vi "add set lengtou2 position(SubVI).vi"(9 "字符串":string) -> (0 "布尔 3":bool, 2 "连接的字符串":string)   [LabVIEW 2019]
panel:
  in  "cancel":bool
  in  "ok":bool
  in  "Position":dbl=2.0 min=0.0 max=400.0
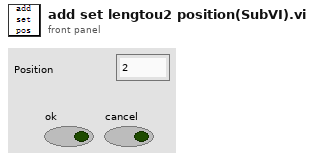
[diagram p1: front panel]
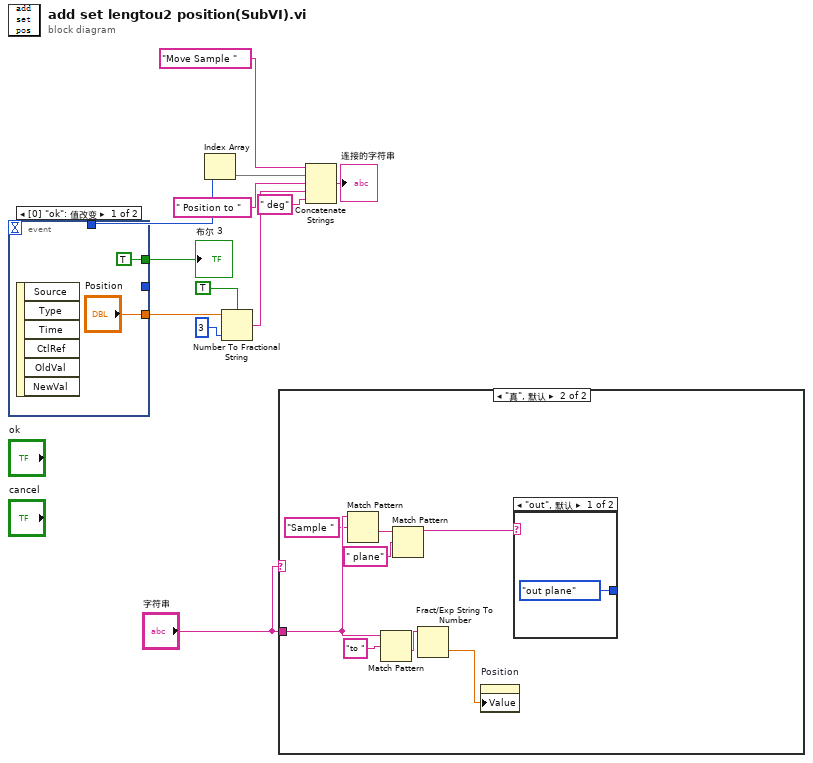
[diagram p0: block diagram]
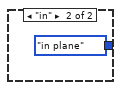
[diagram p3: hidden frame]
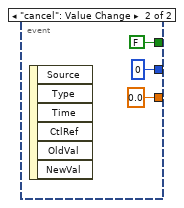
[diagram p4: hidden frame]
diagram:
  n1 = event shown="[0] \"ok\": 值改变" {
    selector: _ -> [_ _]
    dyn-events: _ -> [_ _]
    timeout: _ -> [_ _]
    tunnel: [_ 0 ("Rate输入")] -> _
    tunnel: ["Position" 0.0 ("Field")] -> w12
    tunnel: [TRUE FALSE] -> w13
    tunnel: [w14 _] -> w1
    event "ok": Value Change {
      n2 = event-data() -> ()  [unwired: 1 in, 6 out]
    }
    event "cancel": Value Change {
      n3 = event-data() -> ()  [unwired: 1 in, 6 out]
    }
  }
  "布尔 3" <- w13
  n4 = Index Array(index=w1) -> (array=w6:string[], element=w3)
  n5 = Number To Fractional String(use system decimal point (T)=TRUE ("使用系统小数点(T)"), number=w12, precision (6)=i16 3 ("精度(6)")) -> (F-format string=w10:string)  [unwired: 1 in]
  n6 = case shown="\"真\", 默认" "字符串" {
    tunnel: "字符串" -> [_ w26]
    frame "" {
    }
    frame "真", Default {
      n7 = Match Pattern(string=w26, regular expression="Sample " ("正则表达式")) -> (after substring=w23:string)  [unwired: 1 in, 3 out]
      n8 = Match Pattern(string=w26, regular expression="to " ("正则表达式")) -> (after substring=w28:string)  [unwired: 1 in, 3 out]
      n9 = Match Pattern(string=w23, regular expression=" plane" ("正则表达式")) -> (before substring=w22:string)  [unwired: 1 in, 3 out]
      n10 = Fract/Exp String To Number(string=w28) -> (number=w20:dbl)  [unwired: 3 in, 1 out]
      n11 = property on="Position" class="DigNum (严格)"("Value"=w20) -> ()  [unwired: 2 in, 2 out]
      n12 = case shown="\"out\", 默认" w22 {
        tunnel: [enum16{"in plane", "out plane"}."out plane" ("轴向") enum16{"in plane", "out plane"}."in plane" ("轴向")] -> w21
        frame "out", Default {
        }
        frame "in" {
        }
      }
    }
  }
  n13 = Concatenate Strings("Move Sample " ("字符串"), w3, " Position to ", w10, " deg" ("字符串")) -> (→"连接的字符串":string)
